vi "Proyecto Final.vi"() -> ()   [LabVIEW 2020]
uses:
  <vilib>/Instr/_visa.llb/VISA Configure Serial Port (Instr).vi
panel:
  in  "Activa la Electro-Valvula":bool
  out "Waveform Chart":dbl(graph)
  out "Tank":dbl(slide) scale=0.0..14.0
  out "Litros/Hora":dbl(knob) scale=0.0..500.0
  out "Indicador de Velocidad \nde la Bomba":dbl(knob) scale=0.0..255.0
  out "Confirmación de \nActivación Electro-Valvula":bool
  out "Thermometer":dbl(slide) scale=0.0..50.0
  out "# de caracteres leidos":u32
  out "Terminal Puerto Serier":string
  in  "baud rate (9600)":u32=9600
  in  "VISA resource name":refnum<visa-resource-name>
  in  "stop":bool
  in  "Activa la Bomba":u8(slide) scale=0.0..255.0
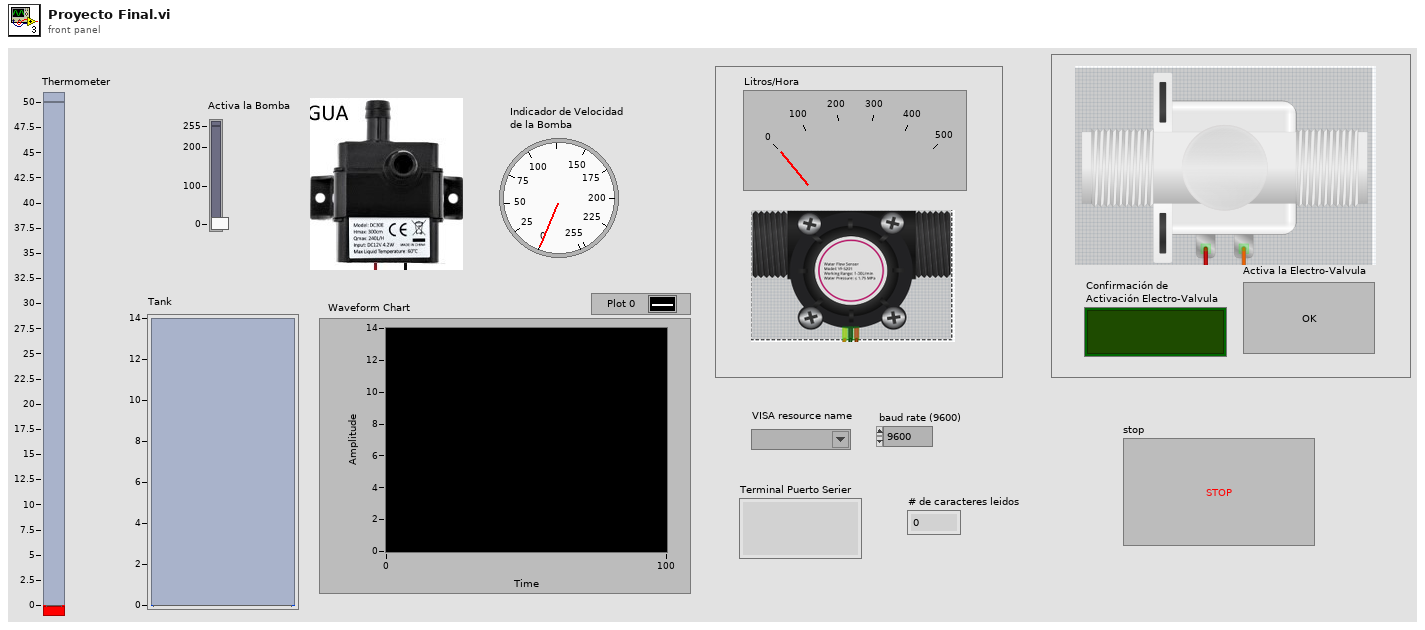
[diagram p1: front panel]
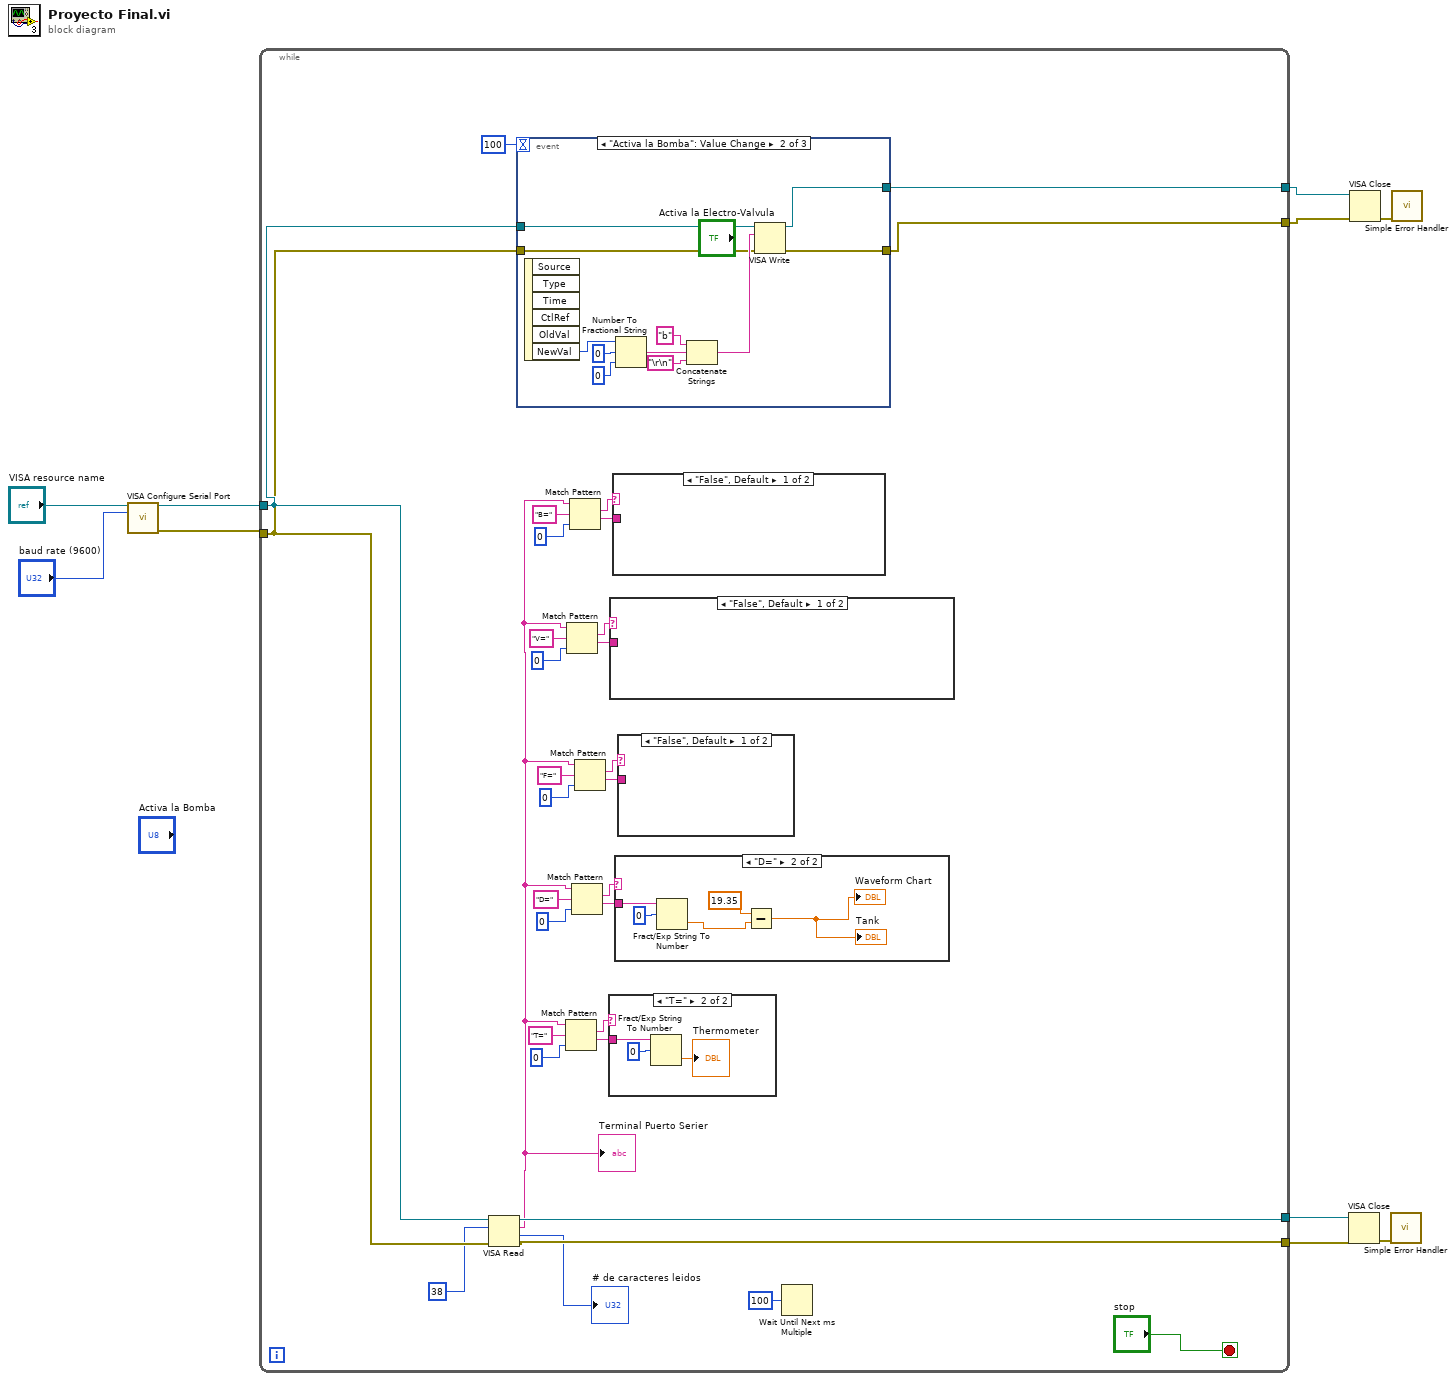
[diagram p0: block diagram]
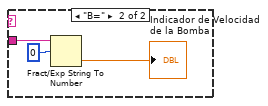
[diagram p2: hidden frame]
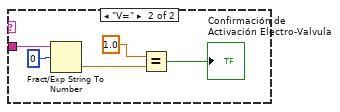
[diagram p3: hidden frame]
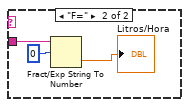
[diagram p4: hidden frame]
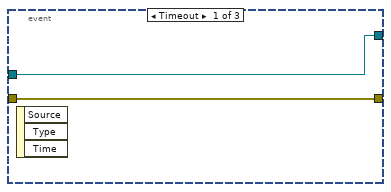
[diagram p7: hidden frame]
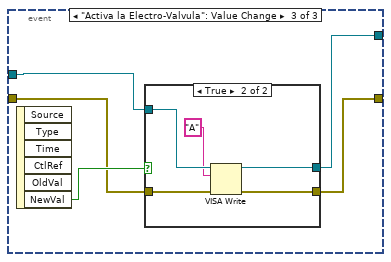
[diagram p8: hidden frame]
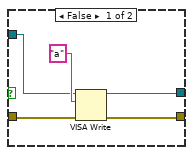
[diagram p9: hidden frame]
diagram:
  n1 = call-poly "VISA Configure Serial Port"("VISA resource name"="VISA resource name", "baud rate (9600)"="baud rate (9600)") -> ("VISA resource name out"=w9:refnum<visa-resource-name>, "error out"=w10:errorcluster)  [unwired: 12 in]
  n2 = while {
    tunnel: w10 -> [w38]
    tunnel: w9 -> [w39]
    tunnel: [w41] -> w6
    tunnel: [w40] -> w5
    tunnel: [w36] -> w2
    tunnel: [w35] -> w1
    stop <- "stop" stop-if-true
    n3 = VISA Read(VISA resource name=w39, byte count=u32 38, error in (no error)=w38) -> (VISA resource name out=w36:refnum<visa-resource-name>, read buffer=w11:string, return count=→"# de caracteres leidos":u32, error out=w35:errorcluster)
    "Terminal Puerto Serier" <- w11
    n4 = event shown="[1] \"Activa la Bomba\": Value Change" {
      selector: _ -> [_ _ _]
      dyn-events: _ -> [_ _ _]
      timeout: 100 -> [_ _ _]
      tunnel: w38 -> [w62 w67 w78]
      tunnel: w39 -> [w63 w66 w77]
      tunnel: [w63 w65 w75] -> w41
      tunnel: [w62 w64 w76] -> w40
      event Timeout {
        n5 = event-data() -> ()  [unwired: 1 in, 3 out]
      }
      event "Activa la Bomba": Value Change {
        n6 = event-data() -> ("NewVal"=w68:u8)  [unwired: 1 in, 5 out]
        n7 = Number To Fractional String(number=w68, width (-)=i16 0, precision (6)=i16 0) -> (F-format string=w70:string)  [unwired: 1 in]
        n8 = Concatenate Strings("b" ("string"), w70, "\r\n") -> (w73:string)
        n9 = VISA Write(VISA resource name=w66, write buffer=w73, error in (no error)=w67) -> (VISA resource name out=w65:refnum<visa-resource-name>, error out=w64:errorcluster)  [unwired: 1 out]
      }
      event "Activa la Electro-Valvula": Value Change {
        n10 = event-data() -> ("NewVal"=w79:bool)  [unwired: 1 in, 5 out]
        n11 = case shown="True" w79 {
          tunnel: w78 -> [w83 w89]
          tunnel: w77 -> [w82 w88]
          tunnel: [w81 w86] -> w76
          tunnel: [w80 w85] -> w75
          frame False {
            n12 = VISA Write(VISA resource name=w82, write buffer="a", error in (no error)=w83) -> (VISA resource name out=w80:refnum<visa-resource-name>, error out=w81:errorcluster)  [unwired: 1 out]
          }
          frame True {
            n13 = VISA Write(VISA resource name=w88, write buffer="A", error in (no error)=w89) -> (VISA resource name out=w85:refnum<visa-resource-name>, error out=w86:errorcluster)  [unwired: 1 out]
          }
        }
      }
    }
    n14 = Match Pattern(string=w11, regular expression="T=", offset (0)=0) -> (match substring=w28:string, after substring=w29:string)  [unwired: 2 out]
    n15 = Match Pattern(string=w11, regular expression="V=", offset (0)=0) -> (match substring=w16:string, after substring=w17:string)  [unwired: 2 out]
    n16 = Match Pattern(string=w11, regular expression="B=", offset (0)=0) -> (match substring=w12:string, after substring=w13:string)  [unwired: 2 out]
    n17 = Match Pattern(string=w11, regular expression="D=", offset (0)=0) -> (match substring=w24:string, after substring=w25:string)  [unwired: 2 out]
    n18 = Match Pattern(string=w11, regular expression="F=", offset (0)=0) -> (match substring=w20:string, after substring=w21:string)  [unwired: 2 out]
    n19 = case shown="\"T=\"" w28 {
      tunnel: w29 -> [_ w60]
      frame "False", Default {
      }
      frame "T=" {
        n20 = Fract/Exp String To Number(string=w60, offset=0) -> (number=→"Thermometer":dbl)  [unwired: 2 in, 1 out]
      }
    }
    n21 = case shown="\"False\", Default" w16 {
      tunnel: w17 -> [_ w49]
      frame "False", Default {
      }
      frame "V=" {
        n22 = Fract/Exp String To Number(string=w49, offset=0) -> (number=w46:dbl)  [unwired: 2 in, 1 out]
        n23 = Equal?(x=1.0, y=w46) -> (x = y?=→"Confirmación de \nActivación Electro-Valvula":bool)
      }
    }
    n24 = case shown="\"False\", Default" w12 {
      tunnel: w13 -> [_ w44]
      frame "False", Default {
      }
      frame "B=" {
        n25 = Fract/Exp String To Number(string=w44, offset=0) -> (number=→"Indicador de Velocidad \nde la Bomba":dbl)  [unwired: 2 in, 1 out]
      }
    }
    n26 = case shown="\"D=\"" w24 {
      tunnel: w25 -> [_ w57]
      frame "False", Default {
      }
      frame "D=" {
        n27 = Fract/Exp String To Number(string=w57, offset=0) -> (number=w56:dbl)  [unwired: 2 in, 1 out]
        n28 = Subtract(x=19.35, y=w56) -> (x-y=→"Tank" →"Waveform Chart":dbl)
      }
    }
    n29 = case shown="\"False\", Default" w20 {
      tunnel: w21 -> [_ w52]
      frame "False", Default {
      }
      frame "F=" {
        n30 = Fract/Exp String To Number(string=w52, offset=0) -> (number=→"Litros/Hora":dbl)  [unwired: 2 in, 1 out]
      }
    }
    n31 = Wait Until Next ms Multiple(millisecond multiple=u32 100) -> ()  [unwired: 1 out]
  }
  n32 = VISA Close(VISA resource name=w2, error in (no error)=w1) -> (error out=w3:errorcluster)
  n33 = VISA Close(VISA resource name=w6, error in (no error)=w5) -> (error out=w4:errorcluster)
  n34 = call <vilib>:"Simple Error Handler.vi"("error in (no error)"=w3) -> ()  [unwired: 4 in, 5 out]
  n35 = call <vilib>:"Simple Error Handler.vi"("error in (no error)"=w4) -> ()  [unwired: 4 in, 5 out]
